vi "TestExec.Funct RTN, Update Local Data.vi"(8 "Error":errorcluster, 10 "RTN Data":T1 {"MeasData"."Status" items=["LOG", "PASS", "FAIL", "ERROR"]; "Attr"."Status" items=["LOG", "PASS", "FAIL", "ERROR"]; "Num"."Status" items=["LOG", "PASS", "FAIL", "ERROR"]}, 11 "Local Data":T1 {"MeasData"."Status" items=["LOG", "PASS", "FAIL", "ERROR"]; "Attr"."Status" items=["LOG", "PASS", "FAIL", "ERROR"]; "Num"."Status" items=["LOG", "PASS", "FAIL", "ERROR"]}) -> (3 "Local Data Out":T1 {"MeasData"."Status" items=["LOG", "PASS", "FAIL", "ERROR"]; "Attr"."Status" items=["LOG", "PASS", "FAIL", "ERROR"]; "Num"."Status" items=["LOG", "PASS", "FAIL", "ERROR"]})   [LabVIEW 2024]
uses:
  TestExec.Local Result Data.ctl
  Results/Result.Attribute.ctl
  Results/Result.Measurement and Attribute Item Status.ctl
  Results/Result.Numeric.ctl
  Results/Result.Limit Type.ctl
  Results/Result XML/TestResult.SW Item.ctl
  Reports/Report.Result FileDataObject.ctl
  Results/Result.Measurement Item.ctl
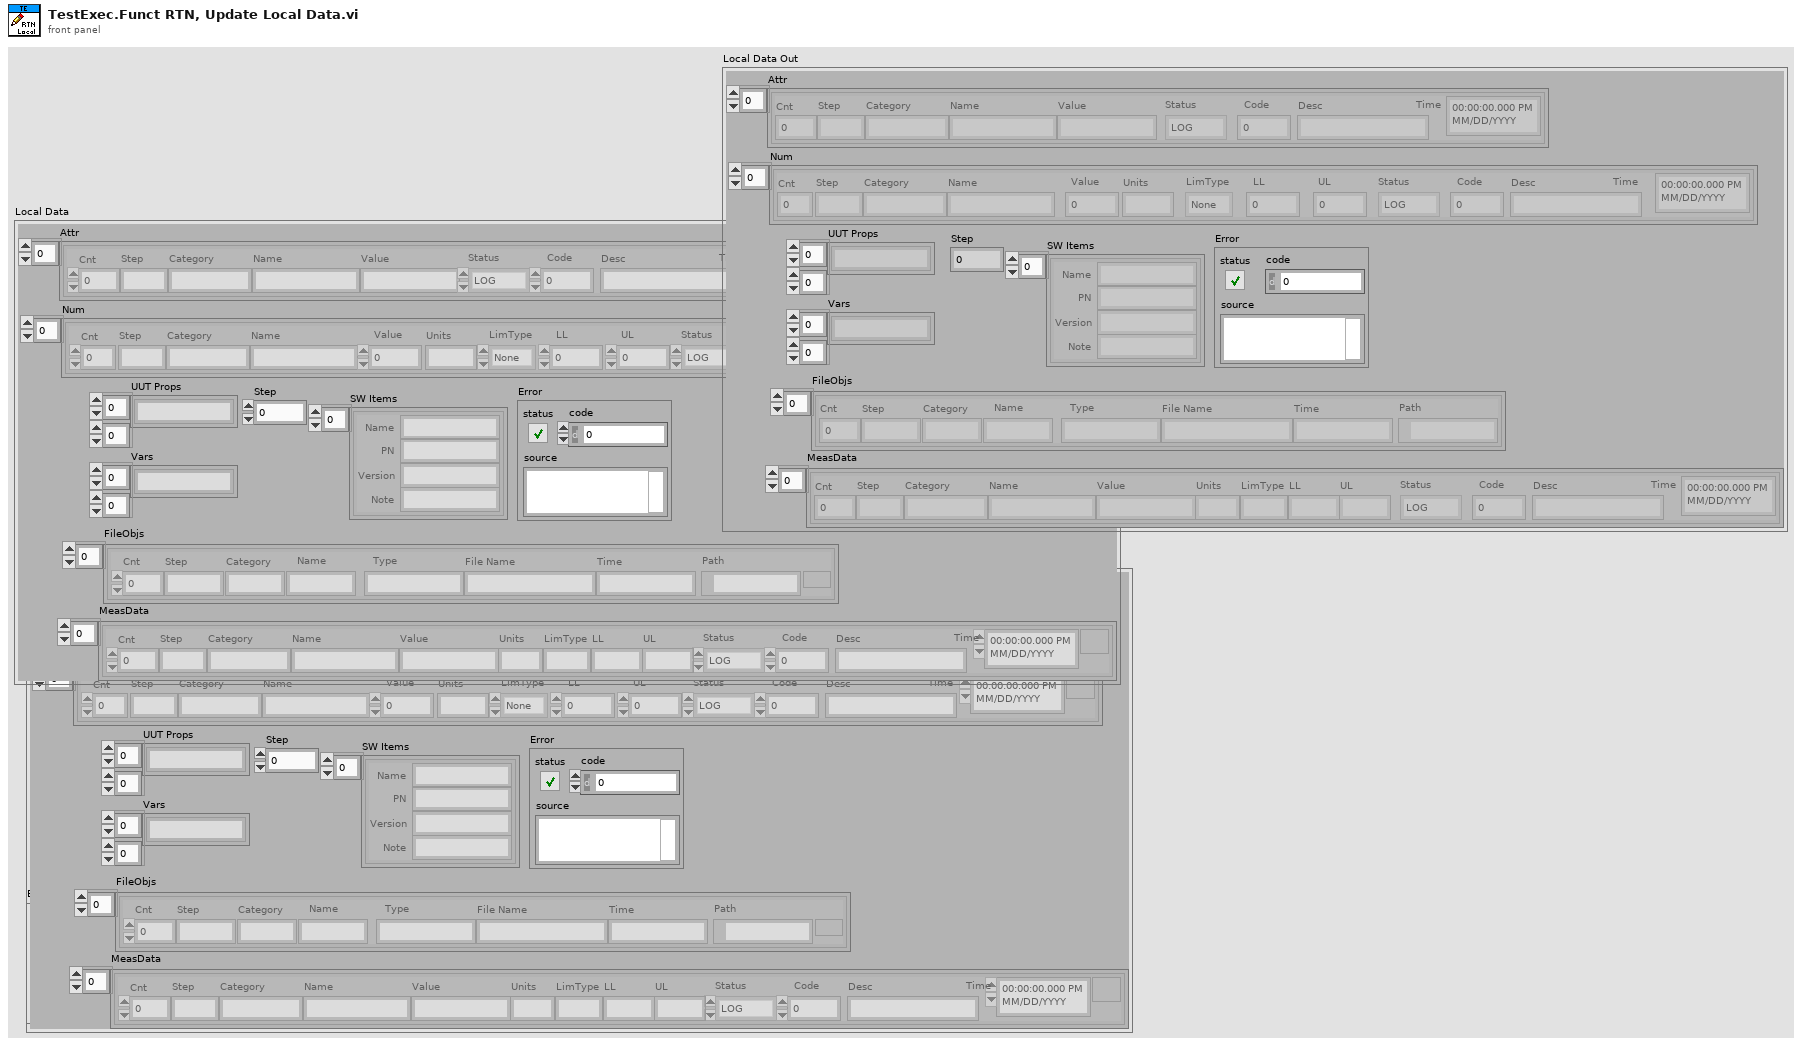
[diagram p1: front panel]
types:
  T1 = typedef "TestExec.Local Result Data.ctl" = cluster{"Attr":T2[], "Num":T4[], "UUT Props":string[][], "Vars":string[][], "SW Items":T6[], "Error":errorcluster, "Step":i32, "FileObjs":T7[], "MeasData":T8[]}
  T2 = typedef "Result.Attribute.ctl" = cluster{"Cnt":i32, "Step":string, "Category":string, "Name":string, "Value":string, "Status":T3, "Code":i32, "Desc":string, "Time":timestamp}
  T3 = typedef "Result.Measurement and Attribute Item Status.ctl" = i32
  T4 = typedef "Result.Numeric.ctl" = cluster{"Cnt":i32, "Step":string, "Category":string, "Name":string, "Value":dbl, "Units":string, "LimType":T5, "LL":dbl, "UL":dbl, "Status":T3, "Code":i32, "Desc":string, "Time":timestamp}
  T5 = typedef "Result.Limit Type.ctl" = enum16{"None", "EQ", "NE", "GT", "LT", "GE", "LE", "GTLT", "GELE", "GELT", "GTLE", "LTGT", "LEGE", "LEGT", "LTGE", "Contains", "NotContains"}
  T6 = typedef "TestResult.SW Item.ctl" = cluster{"Name":string, "PN":string, "Version":string, "Note":string}
  T7 = typedef "Report.Result FileDataObject.ctl" = cluster{"Cnt":i32, "Step":string, "Category":string, "Name":string, "Type":string, "File Name":string, "Time":string, "Path":path}
  T8 = typedef "Result.Measurement Item.ctl" = cluster{"Cnt":i32, "Step":string, "Category":string, "Name":string, "Value":string, "Units":string, "LimType":string, "LL":string, "UL":string, "Status":T3, "Code":i32, "Desc":string, "Time":timestamp}
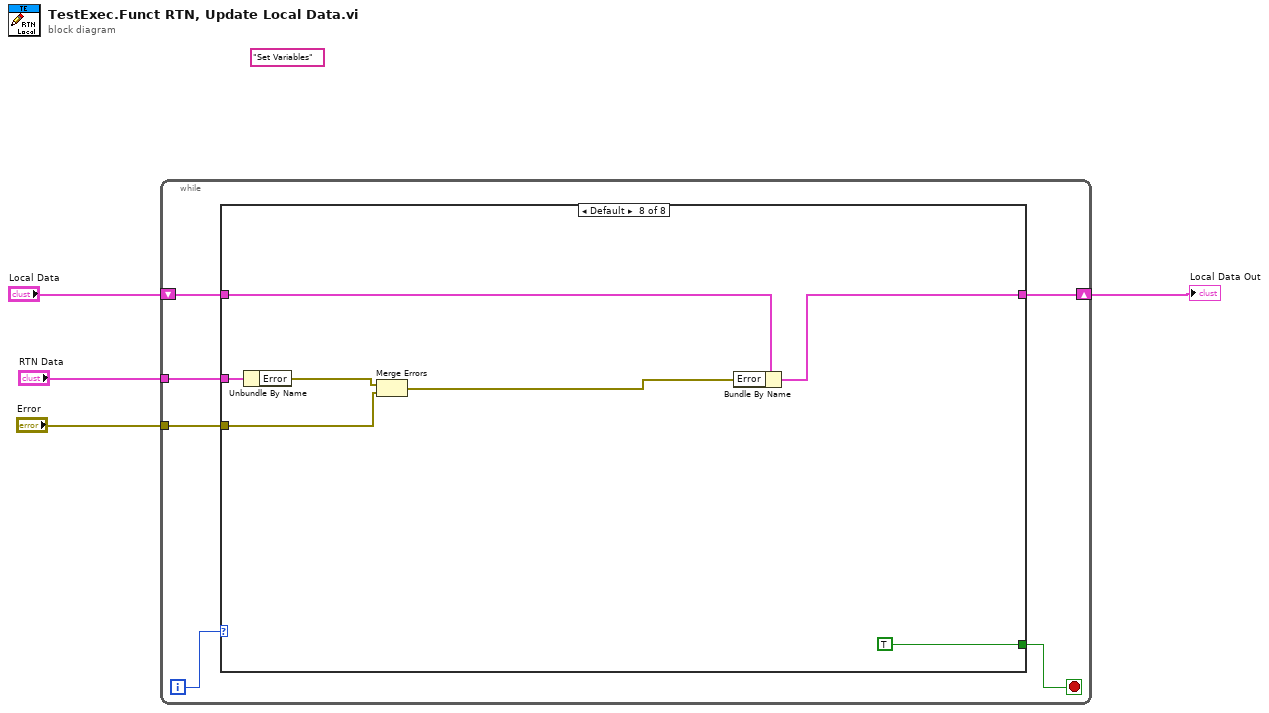
[diagram p0: block diagram]
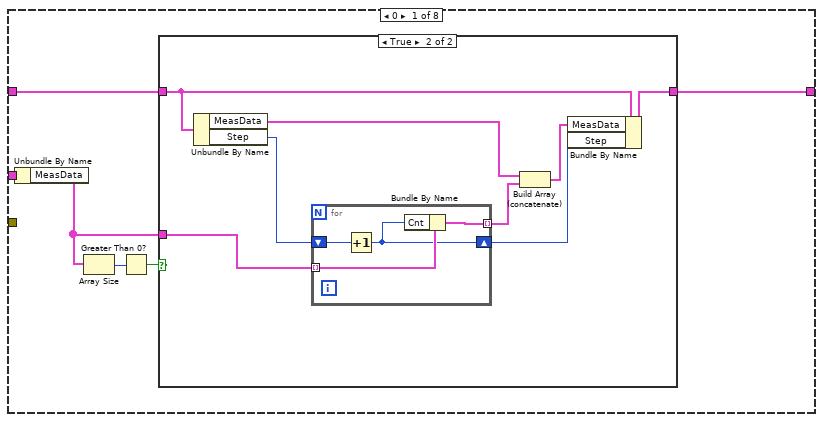
[diagram p2: hidden frame]
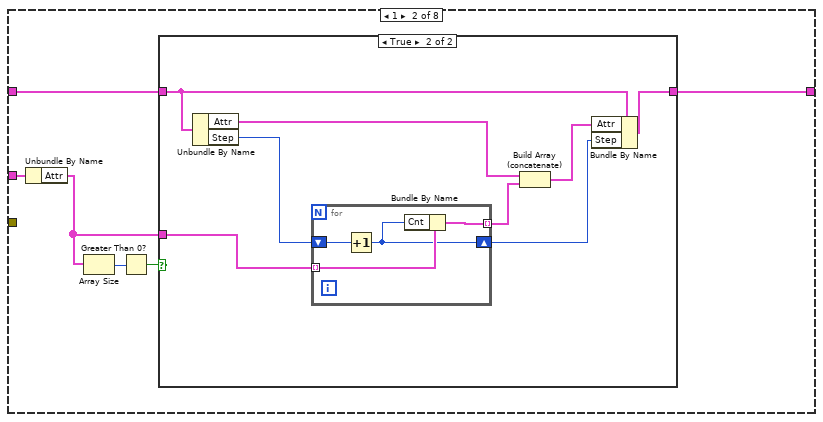
[diagram p4: hidden frame]
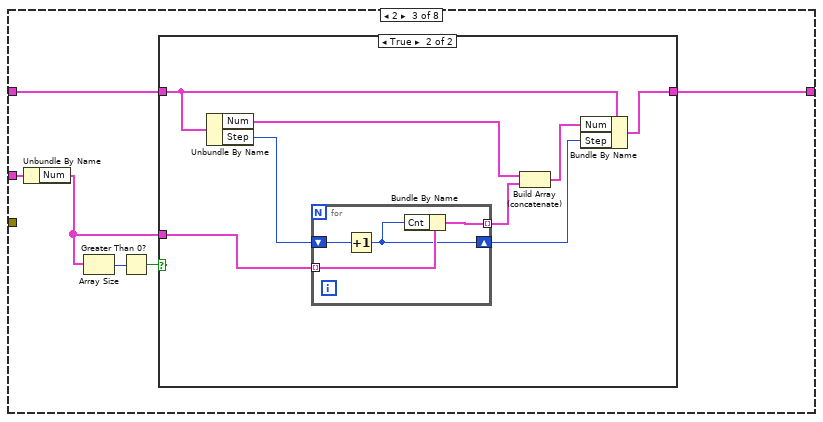
[diagram p6: hidden frame]
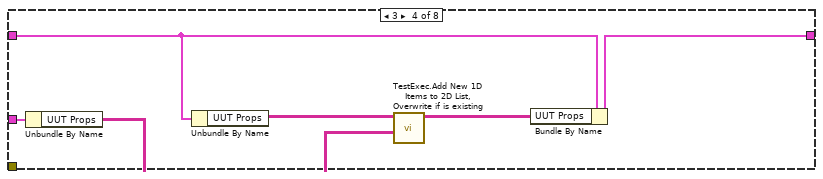
[diagram p8: hidden frame]
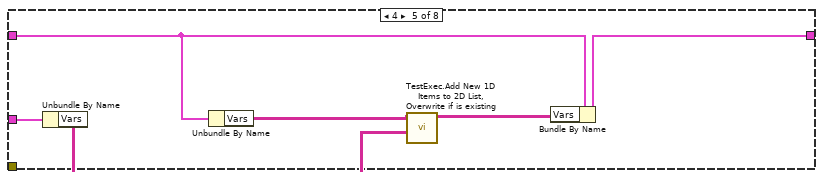
[diagram p9: hidden frame]
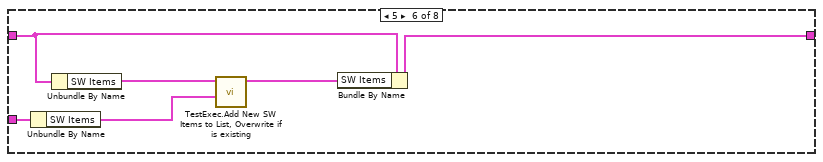
[diagram p10: hidden frame]
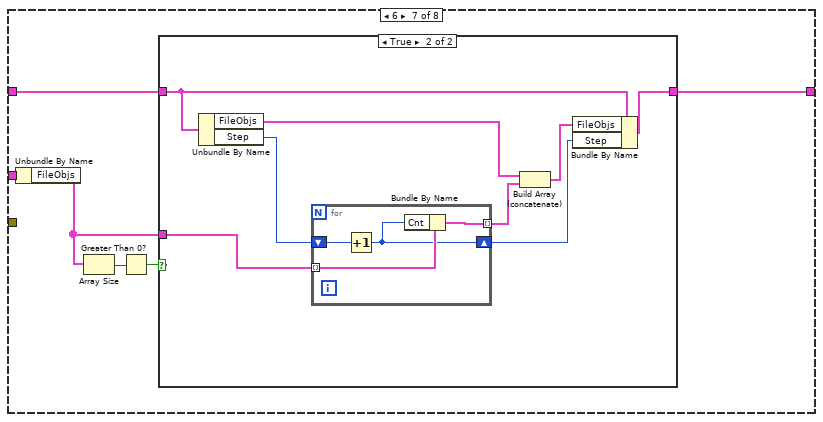
[diagram p11: hidden frame]
diagram:
  (unwired) "Set Variables" ("Cmd")
  n1 = while {
    tunnel: "RTN Data" -> [w8]
    tunnel: "Error" -> [w6]
    shift-right: [w5] -> w1
    shift-left: "Local Data" -> [w7]
    i -> [w10]
    stop <- w9 stop-if-true
    n2 = case shown="Default" w10 {
      tunnel: [_ _ _ _ _ _ _ TRUE] -> w9
      tunnel: w8 -> [w16 w35 w54 w73 w79 w85 w91 w108]
      tunnel: w7 -> [w12 w30 w50 w72 w78 w84 w87 w110]
      tunnel: w6 -> [_ _ _ _ _ _ _ w106]
      tunnel: [w11 w31 w49 w71 w77 w83 w86 w109] -> w5
      frame 0 {
        n3 = Unbundle By Name(w16) -> ("MeasData"=w13:T8[])
        n4 = Array Size(array=w13) -> (size(s)=w14:i32)
        n5 = Greater Than 0?(x=w14) -> (x > 0?=w15:bool)
        n6 = case shown="True" w15 {
          tunnel: w13 -> [_ w20]
          tunnel: w12 -> [w17 w24]
          tunnel: [w17 w21] -> w11
          frame False {
          }
          frame True {
            n7 = Unbundle By Name(w24) -> ("MeasData"=w22:T8[], "Step"=w19:i32)
            n8 = for {
              shift-right: [w26] -> w18
              shift-left: w19 -> [w29]
              tunnel: w20 -> [w28] mode=indexing
              tunnel: [w27] -> w25 mode=indexing
              n9 = Increment(x=w29) -> (x+1=w26:i32)
              n10 = Bundle By Name(cluster=w28, "Cnt"=w26) -> (w27:T8)
            }
            n11 = Build Array (concatenate)(w22, w25) -> (w23:T8[])
            n12 = Bundle By Name(cluster=w24, "MeasData"=w23, "Step"=w18) -> (w21:T1)
          }
        }
      }
      frame 1 {
        n13 = Unbundle By Name(w35) -> ("Attr"=w32:T2[])
        n14 = Array Size(array=w32) -> (size(s)=w33:i32)
        n15 = Greater Than 0?(x=w33) -> (x > 0?=w34:bool)
        n16 = case shown="True" w34 {
          tunnel: w32 -> [_ w39]
          tunnel: w30 -> [w36 w43]
          tunnel: [w36 w40] -> w31
          frame False {
          }
          frame True {
            n17 = Unbundle By Name(w43) -> ("Attr"=w41:T2[], "Step"=w37:i32)
            n18 = for {
              shift-right: [w45] -> w38
              shift-left: w37 -> [w48]
              tunnel: w39 -> [w47] mode=indexing
              tunnel: [w46] -> w44 mode=indexing
              n19 = Increment(x=w48) -> (x+1=w45:i32)
              n20 = Bundle By Name(cluster=w47, "Cnt"=w45) -> (w46:T2)
            }
            n21 = Build Array (concatenate)(w41, w44) -> (w42:T2[])
            n22 = Bundle By Name(cluster=w43, "Attr"=w42, "Step"=w38) -> (w40:T1)
          }
        }
      }
      frame 2 {
        n23 = Unbundle By Name(w54) -> ("Num"=w51:T4[])
        n24 = Array Size(array=w51) -> (size(s)=w52:i32)
        n25 = Greater Than 0?(x=w52) -> (x > 0?=w53:bool)
        n26 = case shown="True" w53 {
          tunnel: w51 -> [_ w58]
          tunnel: w50 -> [w55 w62]
          tunnel: [w55 w59] -> w49
          frame False {
          }
          frame True {
            n27 = Unbundle By Name(w62) -> ("Num"=w60:T4[], "Step"=w57:i32)
            n28 = for {
              shift-right: [w64] -> w56
              shift-left: w57 -> [w67]
              tunnel: w58 -> [w66] mode=indexing
              tunnel: [w65] -> w63 mode=indexing
              n29 = Increment(x=w67) -> (x+1=w64:i32)
              n30 = Bundle By Name(cluster=w66, "Cnt"=w64) -> (w65:T4)
            }
            n31 = Build Array (concatenate)(w60, w63) -> (w61:T4[])
            n32 = Bundle By Name(cluster=w62, "Num"=w61, "Step"=w56) -> (w59:T1)
          }
        }
      }
      frame 3 {
        n33 = Unbundle By Name(w73) -> ("UUT Props"=w69:string[][])
        n34 = Unbundle By Name(w72) -> ("UUT Props"=w70:string[][])
        n35 = call "TestExec.Add New 1D Items to 2D List, Overwrite if is existing.vi"("New Items"=w69, "Item List"=w70) -> ("Item List Out"=w68:string[][])  [unwired: 9 in]
        n36 = Bundle By Name(cluster=w72, "UUT Props"=w68) -> (w71:T1)
      }
      frame 4 {
        n37 = Unbundle By Name(w79) -> ("Vars"=w74:string[][])
        n38 = Unbundle By Name(w78) -> ("Vars"=w76:string[][])
        n39 = call "TestExec.Add New 1D Items to 2D List, Overwrite if is existing.vi"("New Items"=w74, "Item List"=w76) -> ("Item List Out"=w75:string[][])  [unwired: 9 in]
        n40 = Bundle By Name(cluster=w78, "Vars"=w75) -> (w77:T1)
      }
      frame 5 {
        n41 = Unbundle By Name(w85) -> ("SW Items"=w80:T6[])
        n42 = Unbundle By Name(w84) -> ("SW Items"=w82:T6[])
        n43 = call "TestExec.Add New SW Items to List, Overwrite if is existing.vi"("New SW Items"=w80, "SW Items List"=w82) -> ("SW Items List Out"=w81:T6[])  [unwired: 9 in]
        n44 = Bundle By Name(cluster=w84, "SW Items"=w81) -> (w83:T1)
      }
      frame 6 {
        n45 = Unbundle By Name(w91) -> ("FileObjs"=w88:T7[])
        n46 = Array Size(array=w88) -> (size(s)=w89:i32)
        n47 = Greater Than 0?(x=w89) -> (x > 0?=w90:bool)
        n48 = case shown="True" w90 {
          tunnel: w88 -> [_ w95]
          tunnel: w87 -> [w92 w99]
          tunnel: [w92 w96] -> w86
          frame False {
          }
          frame True {
            n49 = Unbundle By Name(w99) -> ("FileObjs"=w97:T7[], "Step"=w94:i32)
            n50 = for {
              shift-right: [w101] -> w93
              shift-left: w94 -> [w104]
              tunnel: w95 -> [w103] mode=indexing
              tunnel: [w102] -> w100 mode=indexing
              n51 = Increment(x=w104) -> (x+1=w101:i32)
              n52 = Bundle By Name(cluster=w103, "Cnt"=w101) -> (w102:T7)
            }
            n53 = Build Array (concatenate)(w97, w100) -> (w98:T7[])
            n54 = Bundle By Name(cluster=w99, "FileObjs"=w98, "Step"=w93) -> (w96:T1)
          }
        }
      }
      frame Default {
        n55 = Unbundle By Name(w108) -> ("Error"=w107:errorcluster)
        n56 = Merge Errors(w107, w106) -> (w105:errorcluster)
        n57 = Bundle By Name(cluster=w110, "Error"=w105) -> (w109:T1)
      }
    }
  }
  "Local Data Out" <- w1
